vi "Teleop.vi"(10 "Match Info":T2={"Autonomous Elapsed Seconds"=0.0, "TeleOp Elapsed Seconds"=0.0, "Disabled Elapsed Seconds"=0.0, "Visited Autonomous"=FALSE, "Visited TeleOp"=FALSE, "Visited Disabled"=FALSE, "Autonomous Settings"={"Autonomous Style"=enum."Independent", "VI Refnum"=refnum}}, 11 "Call Context":T3) -> ()   [LabVIEW 2014]
doc: "This VI is called for each TeleOp packet received from the DS where the robot is not disabled. It is often used to read from the joysticks and update I/O or to update setpoints for timed control loops. It should complete and return within 20 milliseconds or it may miss DS packets."
uses:
  <vilib>/Rock Robotics/WPI/DriverStation/WPI_DriverStationDerivedRobotMode.ctl
  <vilib>/Rock Robotics/WPI/DriverStation/WPI_DriverStationMatch Info.ctl
  <vilib>/Rock Robotics/Network Tables/SD Read Boolean.vi
  <vilib>/Rock Robotics/Network Tables/SD Read Number.vi
  <vilib>/Rock Robotics/WPI/Joystick/WPI_JoystickGetSetRefNum.vi
  <vilib>/Rock Robotics/Network Tables/SD Write Numeric Array.vi
  <vilib>/Rock Robotics/Network Tables/SD Write Boolean Array.vi
  <vilib>/Rock Robotics/WPI/Solenoid/Deprecated/WPI_SolenoidSetBool.vi
panel:
  in  "Enable PIDEnable PIDEnable PIDEnable PIDEnable PIDEnable PID":bool
  out "Btm lim val":bool
  out "top lim val":bool
  out "Toggled Boolean":bool
  in  "Time Since EL actuated":dbl
  in  "Elevator State":bool
  in  "Elevator Locked":bool
  in  "Time Since EJ actuated":dbl
  in  "Ejector State":bool
  in  "time since FG actuated":dbl
  out "Foam Gnome State":bool
  out "axes":T1
  out "Sample Slider 0":dbl(slide) scale=0.0..5.0
  out "Sample Boolean 1":bool
  out "Sample Boolean 0":bool
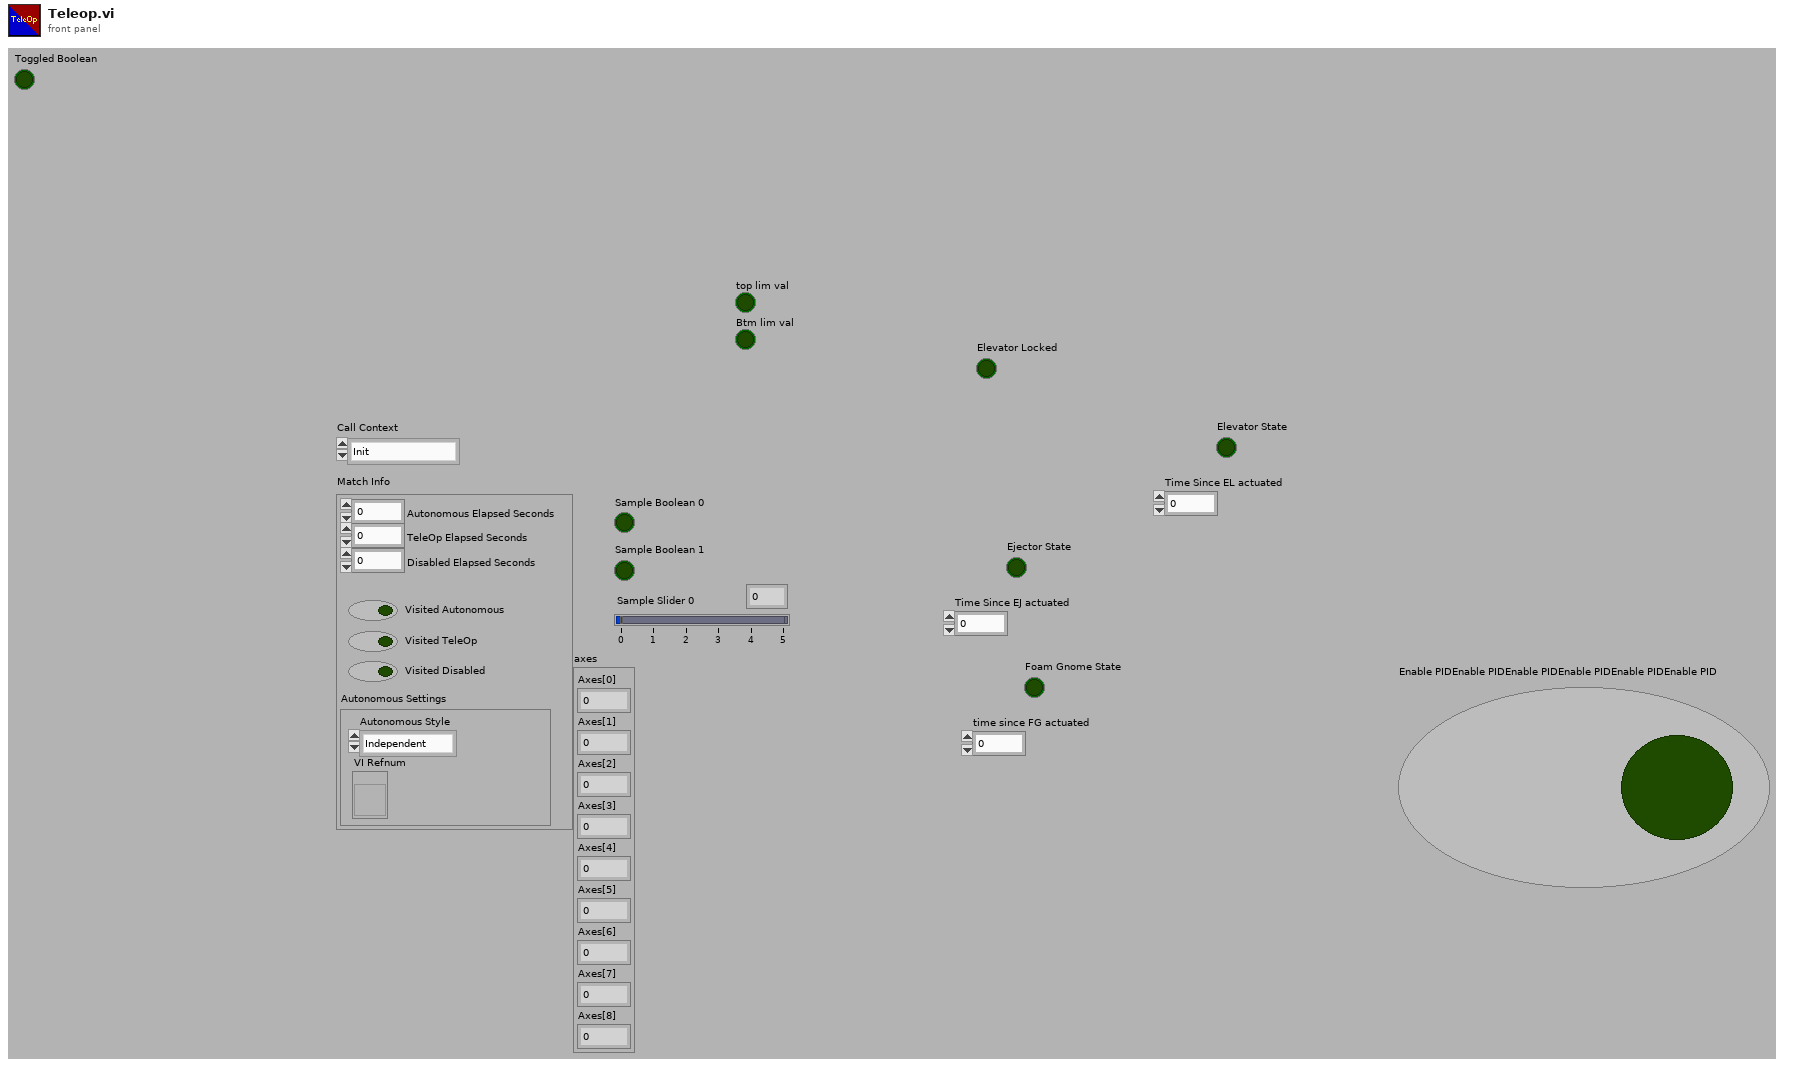
[diagram p1: front panel]
types:
  T1 = cluster{"Axes[0]":dbl, "Axes[1]":dbl, "Axes[2]":dbl, "Axes[3]":dbl, "Axes[4]":dbl, "Axes[5]":dbl, "Axes[6]":dbl, "Axes[7]":dbl, "Axes[8]":dbl}
  T2 = typedef "WPI_DriverStationMatch Info.ctl" = cluster{"Autonomous Elapsed Seconds":dbl, "TeleOp Elapsed Seconds":dbl, "Disabled Elapsed Seconds":dbl, "Visited Autonomous":bool, "Visited TeleOp":bool, "Visited Disabled":bool, "Autonomous Settings":cluster{"Autonomous Style":enum16{"Iterative", "Independent"}, "VI Refnum":refnum<vi>}}
  T3 = typedef "WPI_DriverStationDerivedRobotMode.ctl" = enum16{"Init", "Execute", "Stop"}
  T4 = typedef "WPI_JoystickDevRef.ctl" = cluster{"Device":T5}
  T5 = typedef "WPI_JoystickDeviceEnum.ctl" = enum16{"USB 0", "USB 1", "USB 2", "USB 3", "USB 4", "USB 5"}
  T6 = typedef "WPI_DigitalInputDevRef.ctl" = cluster{"DevStatus":errorcluster, "DIO Channel":T7, "Controller":T8}
  T7 = typedef "FPGA_DIOChannel.ctl" = enum8{"DIO 0", "DIO 1", "DIO 2", "DIO 3", "DIO 4", "DIO 5", "DIO 6", "DIO 7", "DIO 8", "DIO 9", "DIO MXP 0", "DIO MXP 1", "DIO MXP 2", "DIO MXP 3", "DIO MXP 4", "DIO MXP 5", "DIO MXP 6", "DIO MXP 7", "DIO MXP 8", "DIO MXP 9", "DIO MXP 10", "DIO MXP 11", "DIO MXP 12", "DIO MXP 13", "DIO MXP 14", "DIO MXP 15", "Invalid"}
  T8 = typedef "FPGA_TypedefDigitalModule.ctl" = enum16{"Controller 1"}
  T9 = typedef "WPI_MotorControlDeviceRef.ctl" = cluster{"DeviceStatus":errorcluster, "Type":T10, "PWM":cluster{"Controller":T8, "PWM Channel":T11, "DeadBand":T12}, "CAN":cluster{"Device Number":u8, "Control Mode":T13, "Semaphore":T14, "Max Vout":dbl, "TalonSRX Control Mode":T15}, "Invert":bool, "TransformRef":T16, "InvTransformRef":T16}
  T10 = typedef "WPI_MotorControlType.ctl" = enum16{"PWM", "CAN", "CANTalonSRX"}
  T11 = typedef "FPGA_DIOPWMChannel.ctl" = enum8{"PWM 0", "PWM 1", "PWM 2", "PWM 3", "PWM 4", "PWM 5", "PWM 6", "PWM 7", "PWM 8", "PWM 9", "PWM MXP 0", "PWM MXP 1", "PWM MXP 2", "PWM MXP 3", "PWM MXP 4", "PWM MXP 5", "PWM MXP 6", "PWM MXP 7", "PWM MXP 8", "PWM MXP 9", "Invalid"}
  T12 = typedef "WPI_PWMDeadband.ctl" = cluster{"Name":string, "maxPositivePwm":i32, "minPositivePwm":i32, "centerPwm":i32, "maxNegativePwm":i32, "minNegativePwm":i32, "angularRange":u16}
  T13 = typedef "WPI_CANJaguar_ControlMode.ctl" = enum8{"Percent VBus", "Current", "Speed", "Position", "Voltage"}
  T14 = typedef "Semaphore RefNum" = refnum<k1>
  T15 = typedef "WPI_CANTalonSRX_APIControlMode.ctl" = enum8{"Percent VBus", "Speed", "Position", "Slave", "Unchanged / Invalid"}
  T16 = typedef "WPI_PWMTransform_ConPane.ctl" = refnum<vi>
  T17 = typedef "WPI_SolenoidDevRef.ctl" = cluster{"DevStatus":errorcluster, "Pneumatics Control Module":u8, "Forward Solenoid Channel":T18, "Reverse Solenoid Channel":T18}
  T18 = typedef "WPI_SolenoidChannel.ctl" = enum8{"Solenoid 0", "Solenoid 1", "Solenoid 2", "Solenoid 3", "Solenoid 4", "Solenoid 5", "Solenoid 6", "Solenoid 7", "Invalid"}
  T19 = cluster{"Buttons[0]":bool, "Buttons[1]":bool, "Buttons[2]":bool, "Buttons[3]":bool, "Buttons[4]":bool, "Buttons[5]":bool, "Buttons[6]":bool, "Buttons[7]":bool, "Buttons[8]":bool}
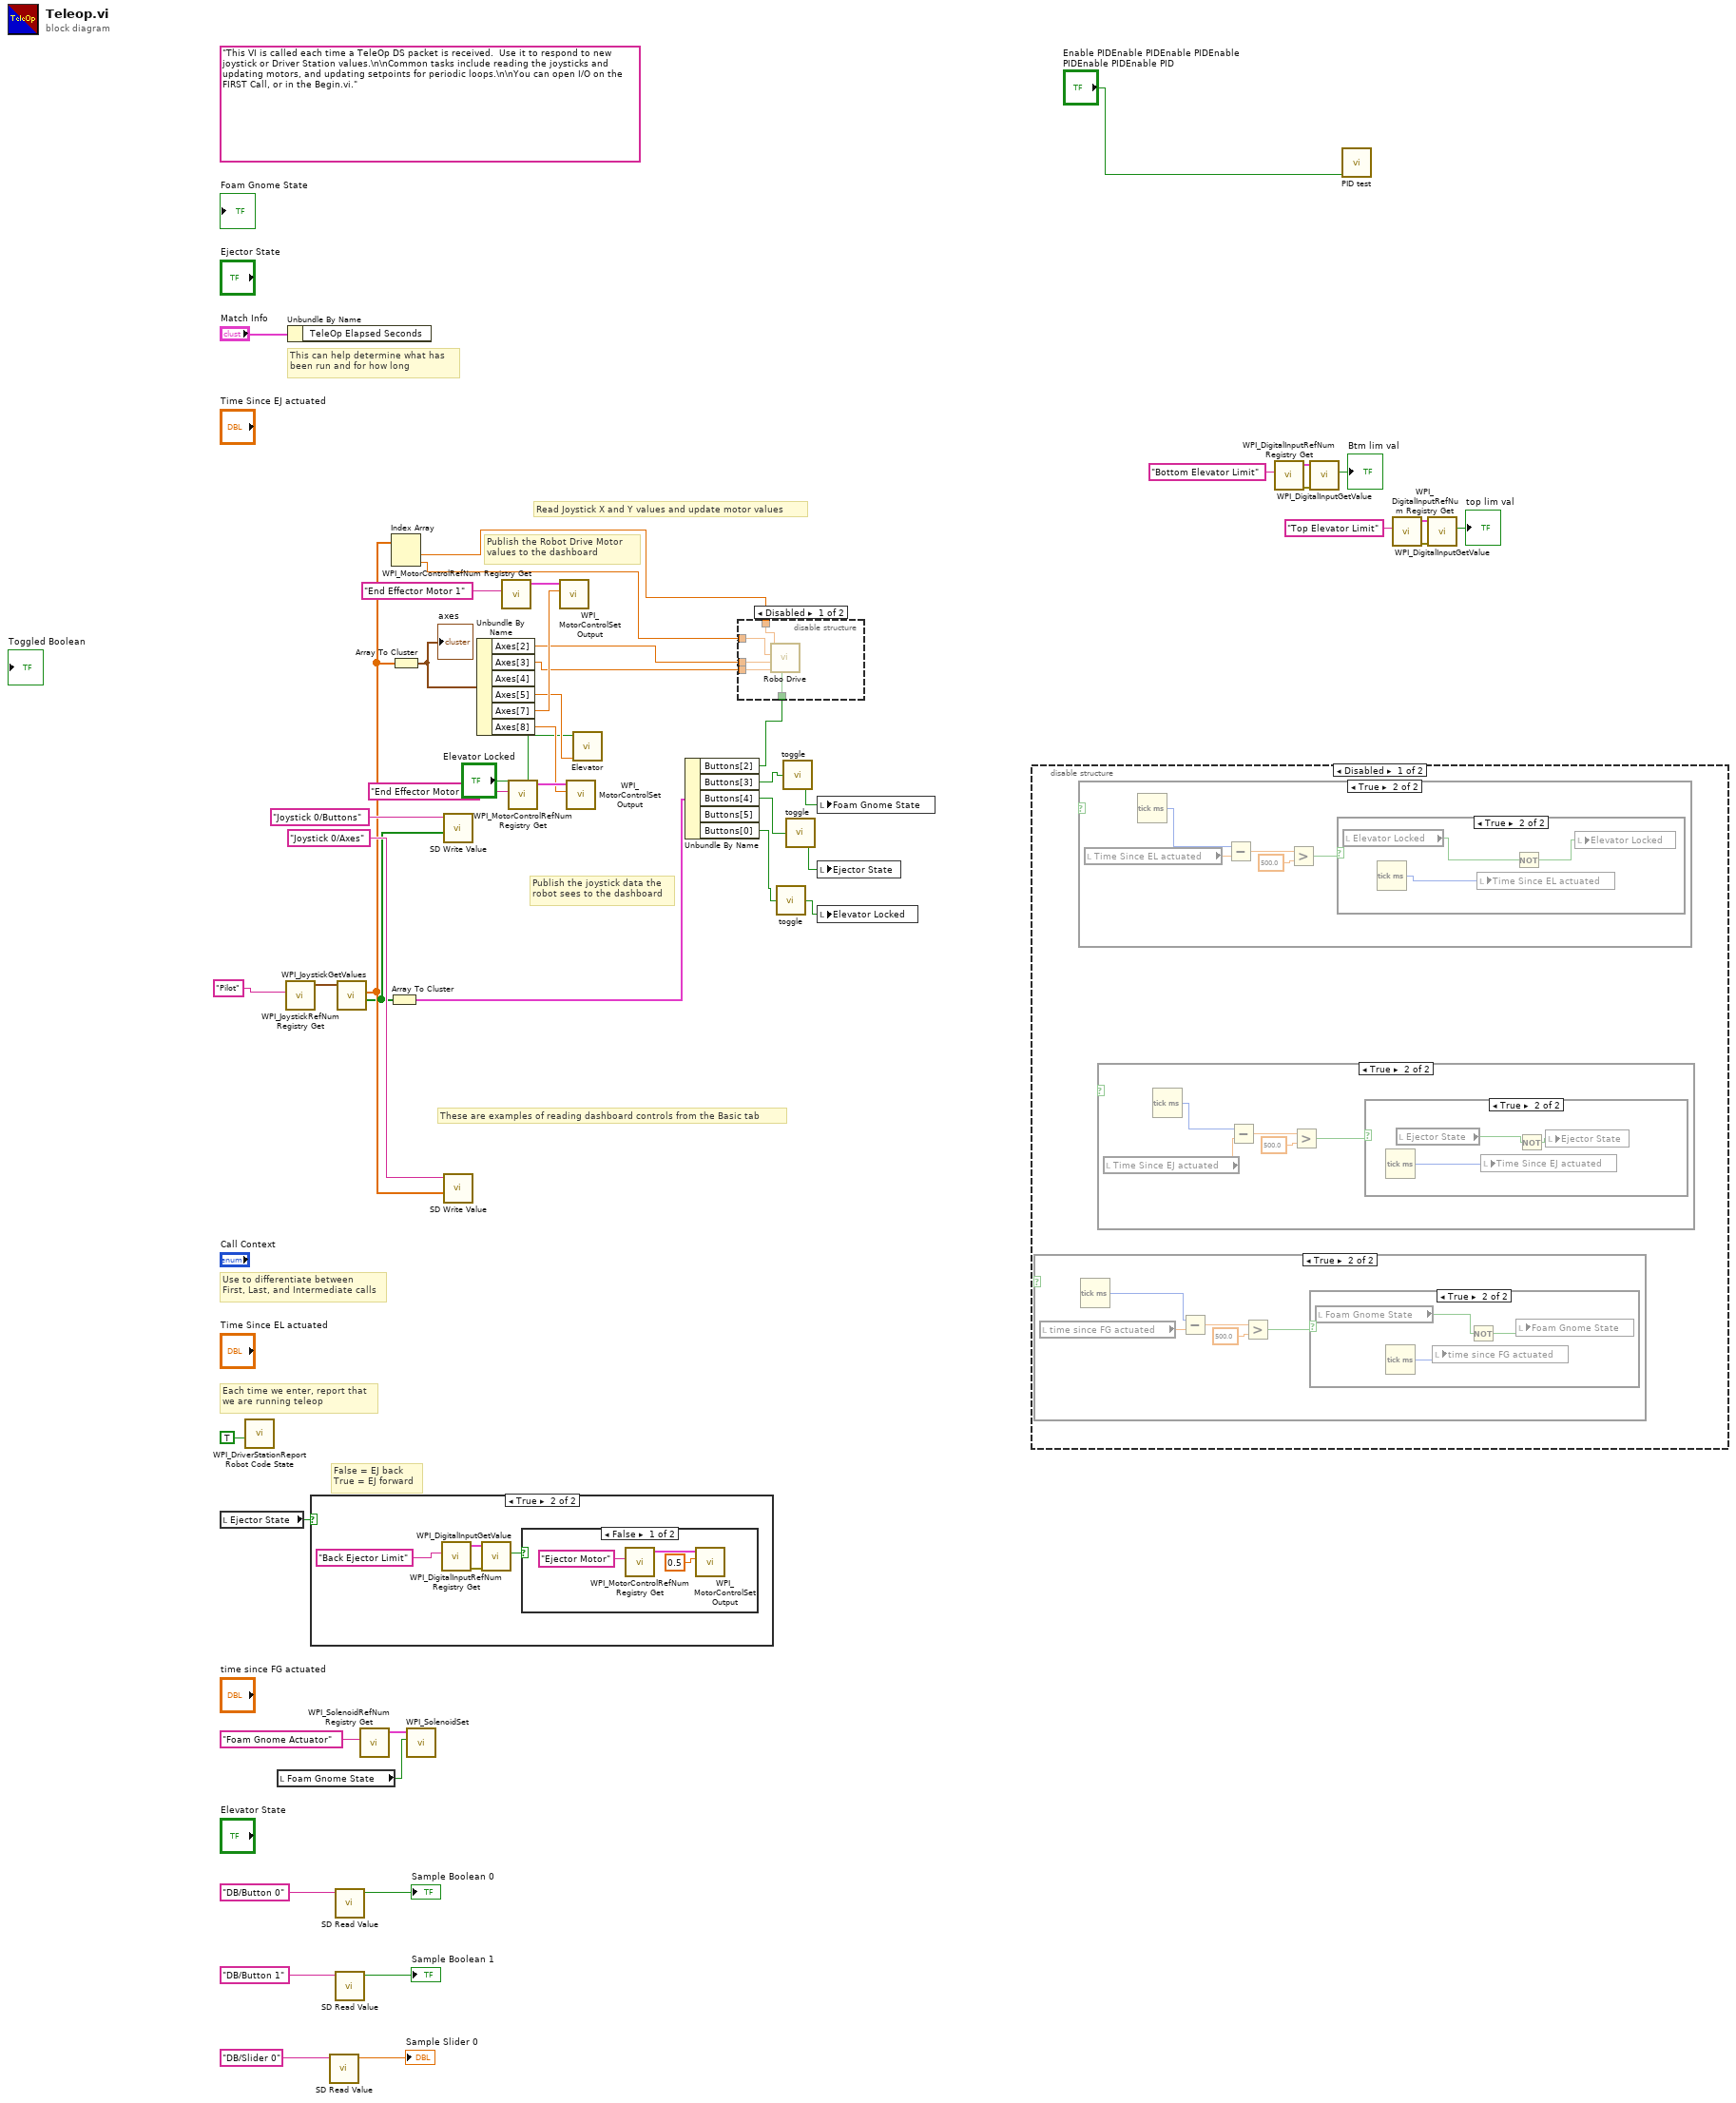
[diagram p0: block diagram]
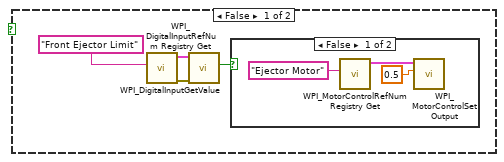
[diagram p10: hidden frame]
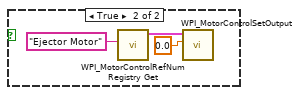
[diagram p11: hidden frame]
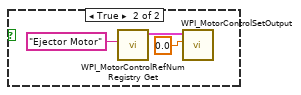
[diagram p12: hidden frame]
diagram:
  (unwired) "This VI is called each time a TeleOp DS packet is received.  Use it to respond to new joystick or Driver Station values.\n\nCommon tasks include reading the joysticks and updating motors, and updating setpoints for periodic loops.\n\nYou can open I/O on the FIRST Call, or in the Begin.vi."
  # "False = EJ back\nTrue = EJ forward"
  # "These are examples of reading dashboard controls from the Basic tab"
  # "Publish the Robot Drive Motor\nvalues to the dashboard"
  # "Publish the joystick data the\nrobot sees to the dashboard"
  # "Each time we enter, report that\nwe are running teleop"
  # "Use to differentiate between\nFirst, Last, and Intermediate calls"
  # "This can help determine what has\nbeen run and for how long"
  # "Read Joystick X and Y values and update motor values"
  n1 = local read "Ejector State"() -> (w24:bool)
  n2 = call <vilib>:"WPI_DriverStationReport Robot Code State.vi"("TeleOp"=TRUE ("Autonomous")) -> ()  [unwired: 10 in, 1 out]
  n3 = local read "Foam Gnome State"() -> (w27:bool)
  n4 = call <vilib>:"WPI_JoystickRefNum Registry Get.vi"("refnum name"="Pilot") -> ("JoystickDevRef"=w47:T4)  [unwired: 1 in, 9 out]
  n5 = Unbundle By Name("Match Info") -> ()  [unwired: 1 out]
  n6 = case shown="True" w24 {
    frame False {
      n7 = call <vilib>:"WPI_DigitalInputRefNum Registry Get.vi"("refnum name"="Front Ejector Limit") -> ("error out"=w52:errorcluster, "DigitalInputDevRef"=w51:T6)  [unwired: 9 in]
      n8 = call <vilib>:"WPI_DigitalInputGetValue.vi"("error in (no error)"=w52, "DigitalInputDevRef"=w51) -> ("Value"=w50:bool)  [unwired: 7 in, 2 out]
      n9 = case shown="False" w50 {
        frame False {
          n10 = call <vilib>:"WPI_MotorControlRefNum Registry Get.vi"("refnum name"="Ejector Motor" ("Name")) -> ("MotorControlDevRef"=w55:T9)  [unwired: 9 in, 1 out]
          n11 = call <vilib>:"WPI_MotorControlSetOutput.vi"("Output"=0.5, "MotorControlDevRef"=w55) -> ()  [unwired: 7 in, 3 out]
        }
        frame True {
          n12 = call <vilib>:"WPI_MotorControlRefNum Registry Get.vi"("refnum name"="Ejector Motor" ("Name")) -> ("MotorControlDevRef"=w58:T9)  [unwired: 9 in, 1 out]
          n13 = call <vilib>:"WPI_MotorControlSetOutput.vi"("Output"=0.0, "MotorControlDevRef"=w58) -> ()  [unwired: 7 in, 3 out]
        }
      }
    }
    frame True {
      n14 = call <vilib>:"WPI_DigitalInputRefNum Registry Get.vi"("refnum name"="Back Ejector Limit") -> ("error out"=w62:errorcluster, "DigitalInputDevRef"=w61:T6)  [unwired: 9 in]
      n15 = call <vilib>:"WPI_DigitalInputGetValue.vi"("error in (no error)"=w62, "DigitalInputDevRef"=w61) -> ("Value"=w60:bool)  [unwired: 7 in, 2 out]
      n16 = case shown="False" w60 {
        frame False {
          n17 = call <vilib>:"WPI_MotorControlRefNum Registry Get.vi"("refnum name"="Ejector Motor" ("Name")) -> ("MotorControlDevRef"=w65:T9)  [unwired: 9 in, 1 out]
          n18 = call <vilib>:"WPI_MotorControlSetOutput.vi"("Output"=0.5, "MotorControlDevRef"=w65) -> ()  [unwired: 7 in, 3 out]
        }
        frame True {
          n19 = call <vilib>:"WPI_MotorControlRefNum Registry Get.vi"("refnum name"="Ejector Motor" ("Name")) -> ("MotorControlDevRef"=w68:T9)  [unwired: 9 in, 1 out]
          n20 = call <vilib>:"WPI_MotorControlSetOutput.vi"("Output"=0.0, "MotorControlDevRef"=w68) -> ()  [unwired: 7 in, 3 out]
        }
      }
    }
  }
  n21 = call-poly <vilib>:"SD Read Value.vi"("Name"="DB/Slider 0" ("refnum name")) -> ("Numeric"=→"Sample Slider 0":dbl)  [unwired: 8 in, 2 out]
  n22 = call-poly <vilib>:"SD Read Value.vi"("Name"="DB/Button 0" ("refnum name")) -> ("Boolean"=→"Sample Boolean 0":bool)  [unwired: 8 in, 2 out]
  n23 = call-poly <vilib>:"SD Read Value.vi"("Name"="DB/Button 1" ("refnum name")) -> ("Boolean"=→"Sample Boolean 1":bool)  [unwired: 8 in, 2 out]
  n24 = call <vilib>:"WPI_JoystickGetValues.vi"("JoystickDevRef"=w47) -> ("Buttons"=w29:bool[], "Axes"=w37:dbl[])  [unwired: 6 in, 3 out]
  n25 = call <vilib>:"WPI_SolenoidRefNum Registry Get.vi"("refnum name"="Foam Gnome Actuator") -> ("SolenoidDevRef"=w31:T17)  [unwired: 9 in, 1 out]
  n26 = Array To Cluster(array=w29) -> (cluster=w28:T19)
  n27 = Index Array(array=w37) -> (element #1=w6:dbl, element #2=w5:dbl)  [unwired: 2 in]
  n28 = Array To Cluster(array=w37) -> (cluster=w36:T1)
  "axes" <- w36
  n29 = call-poly <vilib>:"WPI_SolenoidSet.vi"("Value"=w27, "SolenoidDevRef"=w31) -> ()  [unwired: 8 in, 2 out]
  n30 = call-poly <vilib>:"SD Write Value.vi"("Boolean Array"=w29, "Name"="Joystick 0/Buttons") -> ()  [unwired: 8 in, 2 out]
  n31 = call-poly <vilib>:"SD Write Value.vi"("Numeric Array"=w37, "Name"="Joystick 0/Axes") -> ()  [unwired: 8 in, 2 out]
  n32 = Unbundle By Name(w36) -> ("Axes[2]"=w4:dbl, "Axes[3]"=w3:dbl, "Axes[5]"=w23:dbl, "Axes[7]"=w26:dbl, "Axes[8]"=w25:dbl)  [unwired: 1 out]
  n33 = call <vilib>:"WPI_MotorControlRefNum Registry Get.vi"("refnum name"="End Effector Motor 1" ("Name")) -> ("MotorControlDevRef"=w35:T9)  [unwired: 9 in, 1 out]
  n34 = call <vilib>:"WPI_MotorControlRefNum Registry Get.vi"("refnum name"="End Effector Motor 2" ("Name")) -> ("MotorControlDevRef"=w33:T9)  [unwired: 9 in, 1 out]
  n35 = call <vilib>:"WPI_MotorControlSetOutput.vi"("Output"=w26, "MotorControlDevRef"=w35) -> ()  [unwired: 7 in, 3 out]
  n36 = call <vilib>:"WPI_MotorControlSetOutput.vi"("Output"=w25, "MotorControlDevRef"=w33) -> ()  [unwired: 7 in, 3 out]
  n37 = call "Elevator.vi"("actuating axis"=w23, "Elevator Locked?"="Elevator Locked") -> ()  [unwired: 10 in]
  n38 = Unbundle By Name(w28) -> ("Buttons[2]"=w2:bool, "Buttons[3]"=w17:bool, "Buttons[4]"=w19:bool, "Buttons[0]"=w20:bool)  [unwired: 1 out]
  n39 = disable-structure shown="Disabled" {
    disable-tunnel: w6 -> [w73 _]
    disable-tunnel: w5 -> [w72 _]
    disable-tunnel: w4 -> [w71 _]
    disable-tunnel: w3 -> [w70 _]
    disable-tunnel: w2 -> [w69 _]
    frame Disabled {
      n40 = call "Robo Drive.vi"("Button Flip Directions"=w69, "Right Analog (axes 3)"=w70, "Left Analog (axes 2)"=w71, "Axes 1 (y axis)"=w72, "Axes 0 (x axis)"=w73) -> ()  [unwired: 7 in]
    }
    frame Enabled {
    }
  }
  n41 = call "toggle.vi"("Input"=w20) -> ("Output"=w15:bool)
  n42 = call "toggle.vi"("Input"=w17) -> ("Output"=w16:bool)
  n43 = call "toggle.vi"("Input"=w19) -> ("Output"=w18:bool)
  n44 = local write "Foam Gnome State"(w16) -> ()
  n45 = local write "Ejector State"(w18) -> ()
  n46 = local write "Elevator Locked"(w15) -> ()
  n47 = disable-structure shown="Disabled" {
    frame Disabled {
      n48 = case shown="True" {
        selector: _ -> [_ _]
        frame False {
        }
        frame True {
          n49 = local read "time since FG actuated"() -> (w91:dbl)
          n50 = Tick Count (ms)() -> (millisecond timer value=w90:u32)
          n51 = Subtract(x=w90, y=w91) -> (x-y=w94:dbl)
          n52 = Greater?(x=w94, y=500.0) -> (0:w92:bool)
          n53 = case shown="True" w92 {
            frame False {
            }
            frame True {
              n54 = local read "Foam Gnome State"() -> (w96:bool)
              n55 = Tick Count (ms)() -> (millisecond timer value=w97:u32)
              n56 = local write "time since FG actuated"(w97) -> ()
              n57 = Not(x=w96) -> (.not. x?=w95:bool)
              n58 = local write "Foam Gnome State"(w95) -> ()
            }
          }
        }
      }
      n59 = case shown="True" {
        selector: _ -> [_ _]
        frame False {
        }
        frame True {
          n60 = local read "Time Since EL actuated"() -> (w74:dbl)
          n61 = Tick Count (ms)() -> (millisecond timer value=w75:u32)
          n62 = Subtract(x=w75, y=w74) -> (x-y=w78:dbl)
          n63 = Greater?(x=w78, y=500.0) -> (0:w76:bool)
          n64 = case shown="True" w76 {
            frame False {
            }
            frame True {
              n65 = local read "Elevator Locked"() -> (w81:bool)
              n66 = Tick Count (ms)() -> (millisecond timer value=w79:u32)
              n67 = local write "Time Since EL actuated"(w79) -> ()
              n68 = Not(x=w81) -> (.not. x?=w80:bool)
              n69 = local write "Elevator Locked"(w80) -> ()
            }
          }
        }
      }
      n70 = case shown="True" {
        selector: _ -> [_ _]
        frame False {
        }
        frame True {
          n71 = local read "Time Since EJ actuated"() -> (w82:dbl)
          n72 = Tick Count (ms)() -> (millisecond timer value=w83:u32)
          n73 = Subtract(x=w83, y=w82) -> (x-y=w86:dbl)
          n74 = Greater?(x=w86, y=500.0) -> (0:w84:bool)
          n75 = case shown="True" w84 {
            frame False {
            }
            frame True {
              n76 = Tick Count (ms)() -> (millisecond timer value=w87:u32)
              n77 = local read "Ejector State"() -> (w89:bool)
              n78 = local write "Time Since EJ actuated"(w87) -> ()
              n79 = Not(x=w89) -> (.not. x?=w88:bool)
              n80 = local write "Ejector State"(w88) -> ()
            }
          }
        }
      }
    }
    frame Enabled {
    }
  }
  n81 = call <vilib>:"WPI_DigitalInputRefNum Registry Get.vi"("refnum name"="Bottom Elevator Limit") -> ("error out"=w10:errorcluster, "DigitalInputDevRef"=w9:T6)  [unwired: 9 in]
  n82 = call <vilib>:"WPI_DigitalInputGetValue.vi"("error in (no error)"=w10, "DigitalInputDevRef"=w9) -> ("Value"=→"Btm lim val":bool)  [unwired: 7 in, 2 out]
  n83 = call "PID test.vi"("Enable PID"="Enable PIDEnable PIDEnable PIDEnable PIDEnable PIDEnable PID") -> ()  [unwired: 11 in]
  n84 = call <vilib>:"WPI_DigitalInputRefNum Registry Get.vi"("refnum name"="Top Elevator Limit") -> ("error out"=w14:errorcluster, "DigitalInputDevRef"=w13:T6)  [unwired: 9 in]
  n85 = call <vilib>:"WPI_DigitalInputGetValue.vi"("error in (no error)"=w14, "DigitalInputDevRef"=w13) -> ("Value"=→"top lim val":bool)  [unwired: 7 in, 2 out]
